vi "DAQmxTaskContainerUpdate-Com-Exec.vi"(8 "error in (no error)":errorcluster, 9 "data":variant, 11 "DAQmxTaksContainer_General in":refnum<class "DAQmxTaksContainer_General.lvclass">) -> (0 "error out":errorcluster, 3 "DAQmxTaksContainer_General out":refnum<class "DAQmxTaksContainer_General.lvclass">)   [LabVIEW 2018, in "DAQmxTaksContainer_General.lvclass"]
uses:
  DAQmxTaksContainer_General.lvclass
  C:/Users/Sergey Denisov/Documents/REPS/TRANCON/Classes/GeneralFunctionality/GeneralFunctionality.lvclass
  GeneralFunctionality/GeneralFunctionality.lvclass/GeneralFunctionality.ctl
  Config/Config.lvclass/Config.ctl
  DAQmxTaksContainer_General.lvclass/DAQmxTaksContainer_General.ctl
  Config/Config.lvclass
  DAQmxTask.lvclass
  GeneralFunctionality/GeneralFunctionality.lvclass
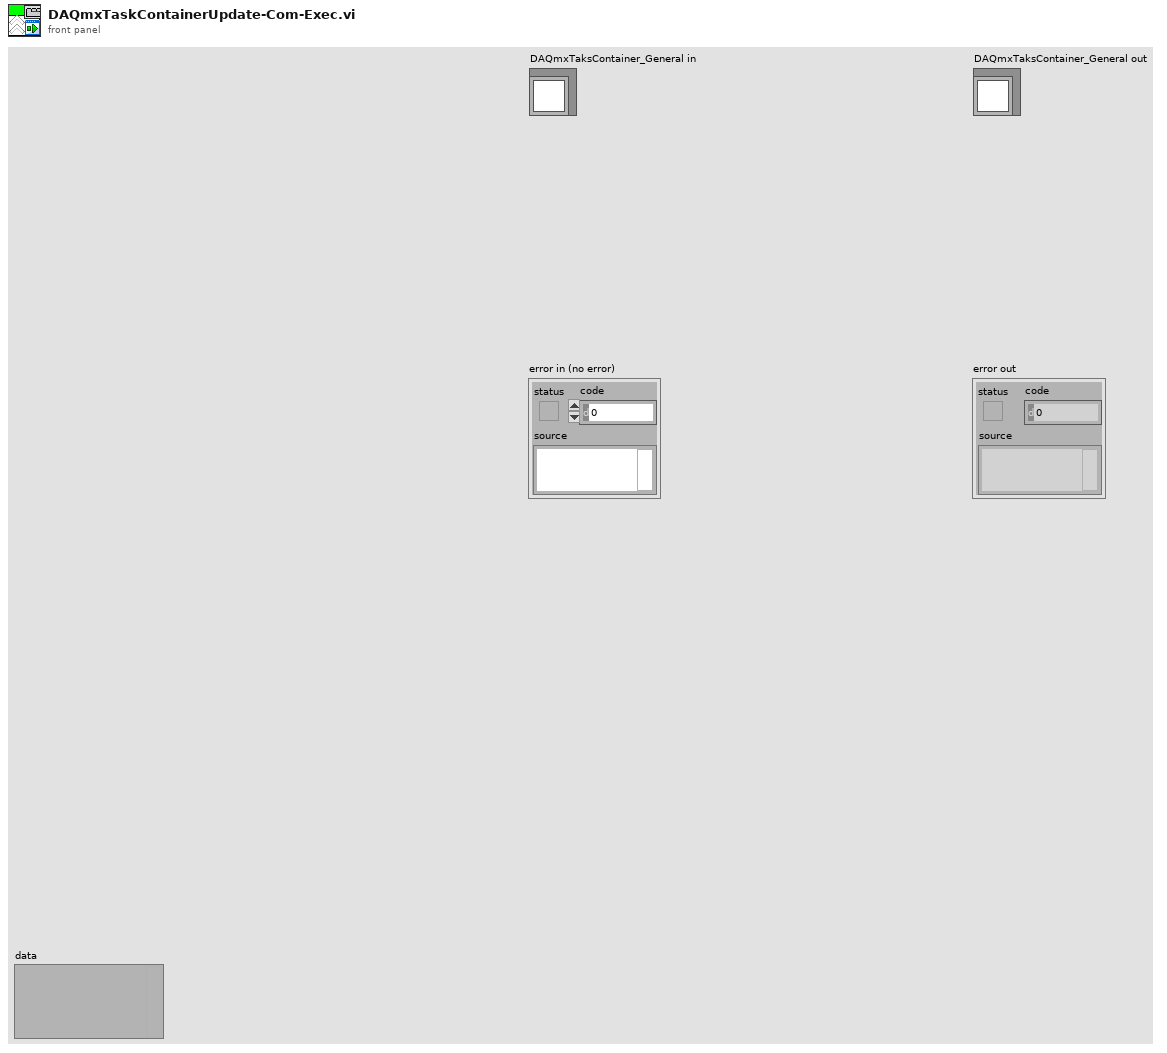
[diagram p1: front panel]
types:
  T1 = enum8{"Enabled", "Disabled", "Disabled and Grayed Out"}
  T2 = cluster{"name":string, "type of task":string, "Status":bool, "Value":string, "error":errorcluster}
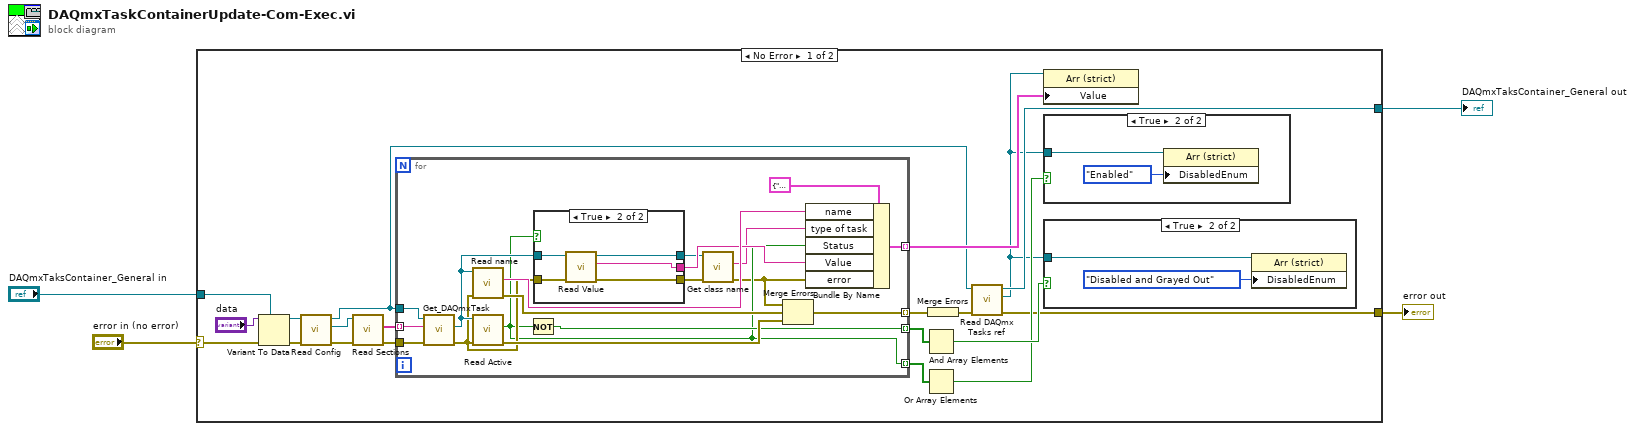
[diagram p0: block diagram]
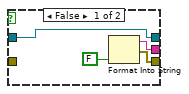
[diagram p4: hidden frame]
diagram:
  n1 = case shown="No Error" "error in (no error)" {
    selector: "error in (no error)" -> [w10 w57]
    tunnel: "DAQmxTaksContainer_General in" -> [w24 w56]
    tunnel: [w8 w57] -> w4
    tunnel: [w6 w56] -> w3
    frame No Error {
      n2 = Variant To Data(error in=w10, type=w24, Variant="data") -> (data=w13:refnum<class "DAQmxTaksContainer_General.lvclass">, error out=w12:errorcluster)
      n3 = call "Read Config.vi"("error in (no error)"=w12, "GeneralFunctionality en entrée"=w13) -> ("error out"=w22:errorcluster, "Config.lvclass"=w21:refnum<class "Config.lvclass">, "GeneralFunctionality en sortie"=w7:refnum<class "DAQmxTaksContainer_General.lvclass">)  [unwired: 7 in]
      n4 = call "Read Sections.vi"("error in (no error)"=w22, "Config in"=w21) -> ("error out"=w19:errorcluster, "Sections"=w20:string[])  [unwired: 7 in, 1 out]
      n5 = for {
        tunnel: w7 -> [w46]
        tunnel: w20 -> [w45] mode=indexing
        tunnel: w19 -> [w44]
        tunnel: [w38] -> w18 mode=indexing
        tunnel: [w37] -> w11 mode=indexing
        tunnel: [w31] -> w17 mode=indexing
        tunnel: [w30] -> w15 mode=indexing
        n6 = call "Get_DAQmxTask.vi"("error in (no error)"=w44, "Task name"=w45, "DAQmxTaksContainer_General in"=w46) -> ("error out"=w35:errorcluster, "DAQmx Task"=w36:refnum<class "DAQmxTask.lvclass">)  [unwired: 6 in, 1 out]
        n7 = call "Read name.vi"("error in (no error)"=w35, "DAQmxTask in"=w36) -> ("error out"=w39:errorcluster, "name"=w42:string)  [unwired: 7 in, 1 out]
        n8 = call-dynamic "Read Active.vi"("error in (no error)"=w35, "DAQmxTask in"=w36) -> ("error out"=w40:errorcluster, "Active?"=w30:bool)  [unwired: 7 in, 1 out]
        n9 = Not(x=w30) -> (.not. x?=w31:bool)
        n10 = case shown="True" w30 {
          tunnel: [w49 w52] -> w41
          tunnel: [w50 w53] -> w33
          tunnel: w36 -> [w47 w55]
          tunnel: w35 -> [_ w54]
          tunnel: [w47 w51] -> w34
          frame False {
            n11 = Format Into String(FALSE ("input 1")) -> (resulting string=w49:string, error out=w50:errorcluster)  [unwired: 3 in]
          }
          frame True {
            n12 = call-dynamic "Read Value.vi"("error in (no error)"=w54, "DAQmxTask en entrée"=w55) -> ("error out"=w53:errorcluster, "Data string"=w52:string, "DAQmxTask en sortie"=w51:refnum<class "DAQmxTask.lvclass">)  [unwired: 6 in, 1 out]
          }
        }
        n13 = call "Get class name.vi"("error in (no error)"=w33, "DAQmxTask en entrée"=w34) -> ("error out"=w29:errorcluster, "Class name"=w32:string)  [unwired: 7 in, 1 out]
        n14 = Merge Errors(w29, w39, w40) -> (w38:errorcluster)
        n15 = Bundle By Name(cluster=T2 {"name"="", "type of task"="", "Status"=FALSE, "Value"="", "error"={"status"=FALSE, "code"=0, "source"=""}} ("Task"), "name"=w42, "type of task"=w32, "Status"=w30, "Value"=w41, "error"=w29) -> (w37:T2)
      }
      n16 = And Array Elements(Boolean array=w17) -> (logical AND=w16:bool)
      n17 = Or Array Elements(Boolean array=w15) -> (logical OR=w14:bool)
      n18 = Merge Errors(w18) -> (w9:errorcluster)
      n19 = call "Read DAQmx Tasks ref.vi"("error in (no error)"=w9, "DAQmxTaksContainer_General in"=w7) -> ("error out"=w8:errorcluster, "DAQmx Tasks ref"=w5:refnum<vi>, "DAQmxTaksContainer_General out"=w6:refnum<class "DAQmxTaksContainer_General.lvclass">)  [unwired: 7 in]
      n20 = property class="Arr (strict)"(reference=w5, "Value"=w11) -> ()  [unwired: 1 in, 2 out]
      n21 = case shown="True" w14 {
        tunnel: w5 -> [_ w25]
        frame False {
        }
        frame True {
          n22 = property class="Arr (strict)"(reference=w25, "DisabledEnum"=T1."Enabled" ("Désactivé")) -> ()  [unwired: 1 in, 2 out]
        }
      }
      n23 = case shown="True" w16 {
        tunnel: w5 -> [_ w28]
        frame False {
        }
        frame True {
          n24 = property class="Arr (strict)"(reference=w28, "DisabledEnum"=T1."Disabled and Grayed Out" ("Désactivé")) -> ()  [unwired: 1 in, 2 out]
        }
      }
    }
    frame Error {
    }
  }
  "error out" <- w4
  "DAQmxTaksContainer_General out" <- w3
